vi "Sense.vi"(2 "World":i8[][](array[numeric]), 3 "Y":i8, 4 "X":i8) -> (0 "Heading":i8, 1 "Sensor Array":i8[][](array[numeric]))   [LabVIEW 2014]
doc: "This VI returns a 3x3 subsection of the world array and the direction of the highest value neighbor based on the V code key. If there is no highest-valued neighbor, it returns a random number from 1 to 8.\n\nV code\n 6 7 8\n 5 0 1\n 4 3 2"
panel:
  # "Vcode\n  6 7 8\n  5 0 1\n  4 3 2"
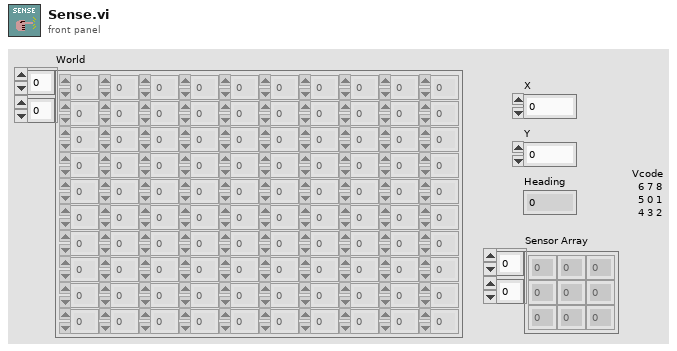
[diagram p1: front panel]
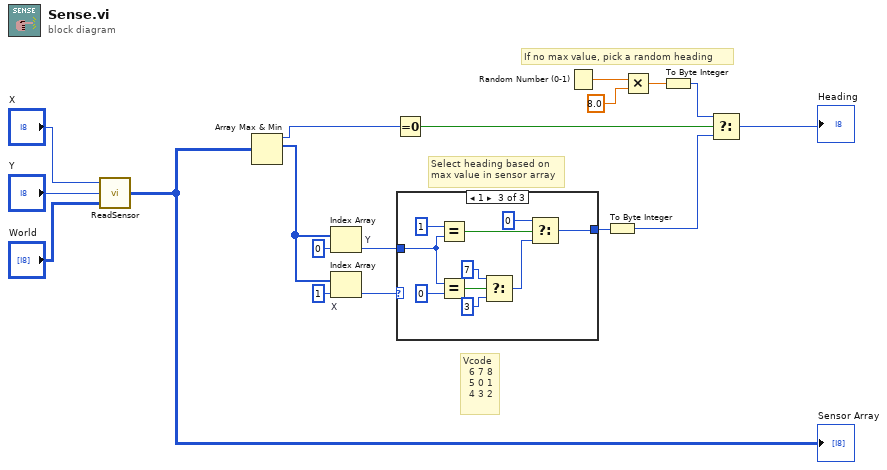
[diagram p0: block diagram]
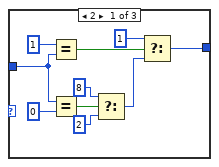
[diagram p2: hidden frame]
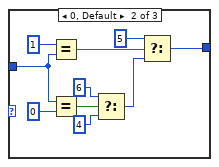
[diagram p3: hidden frame]
diagram:
  # "If no max value, pick a random heading"
  # "Select heading based on\nmax value in sensor array"
  # "Vcode\n  6 7 8\n  5 0 1\n  4 3 2"
  n1 = call "ReadSensor.vi"("World"="World", "Y"="Y", "X"="X") -> ("Sensor Array"=w6:i8[][])
  "Sensor Array" <- w6
  n2 = Array Max & Min(array=w6) -> (max value=w15:i8, max index (indices)=w9:i32[])  [unwired: 2 out]
  n3 = Index Array "Y"(array=w9, index=0) -> (element=w7:i32)
  n4 = Index Array "X"(array=w9, index=1) -> (element=w8:i32)
  n5 = Equal To 0?(x=w15) -> (x = 0?=w14:bool)
  n6 = case shown="1" w8 {
    tunnel: w7 -> [w28 w38 w48]
    tunnel: [w23 w33 w43] -> w5
    frame 2 {
      n7 = Equal?(x=1, y=w28) -> (x = y?=w25:bool)
      n8 = Equal?(x=w28, y=0) -> (x = y?=w24:bool)
      n9 = Select(t=8 ("y"), s=w24, f=2 ("y")) -> (s? t:f=w20:i32)
      n10 = Select(t=1, s=w25, f=w20) -> (s? t:f=w23:i32)
    }
    frame 0, Default {
      n11 = Equal?(x=1, y=w38) -> (x = y?=w35:bool)
      n12 = Equal?(x=w38, y=0) -> (x = y?=w34:bool)
      n13 = Select(t=6 ("y"), s=w34, f=4 ("y")) -> (s? t:f=w30:i32)
      n14 = Select(t=5, s=w35, f=w30) -> (s? t:f=w33:i32)
    }
    frame 1 {
      n15 = Equal?(x=1, y=w48) -> (x = y?=w45:bool)
      n16 = Equal?(x=w48, y=0) -> (x = y?=w44:bool)
      n17 = Select(t=7 ("y"), s=w44, f=3 ("y")) -> (s? t:f=w40:i32)
      n18 = Select(t=0, s=w45, f=w40) -> (s? t:f=w43:i32)
    }
  }
  n19 = Random Number (0-1)() -> (number: 0 to 1=w2:dbl)
  n20 = To Byte Integer(number=w5) -> (8bit integer=w4:i8)
  n21 = Multiply(x=w2, y=8.0) -> (x*y=w3:dbl)
  n22 = To Byte Integer(number=w3) -> (8bit integer=w12:i8)
  n23 = Select(t=w12, s=w14, f=w4) -> (s? t:f=→"Heading":i8)
